vi "rszvl_core_global.vi"() -> ()   [LabVIEW 2014] (continued)
 BTO Get Modulation Accuracy of DEVM 99%:\nThis attribute reads the 99% of differential error vector magnitude (DEVM) in the Carrier Frequency Stability and Modulation Accuracy measurement.\n\nNote:\n\n(1) This command is only available with active Carrier Frequency Stability and Modulation\nAccuracy measurement.\n\n(18) BTO Get Carrier Frequency Stability Total Frequency Error Value:\nThis attribute reads the value of carrier frequency deviation of all packets in the Carrier Frequency Stability and Modulation Accuracy measurement.\n\nNote(s):\n\n(1) This command is only available with active Carrier Frequency Stability and Modulation Accuracy measurement\n\n(19) BTO Get Carrier Frequency Stability Block Frequency Error Value:\nThis attribute reads the frequency deviation of all blocks in the Carrier Frequency Stability and Modulation Accuracy measurement.\n\nNote(s):\n\n(1) This command is only available with active Carrier Frequency Stability and Modulation Accuracy measurement\n\n(20) BTO Get Carrier Frequency Stability Initial Frequency Error Value:\nThis attribute reads the combined frequency deviation of all packets and all blocks in the Carrier Frequency Stability and Modulation Accuracy measurement.\n\nNote(s):\n\n(1) This command is only available with active Carrier Frequency Stability and Modulation Accuracy measurement\n\n(21) BTO Get Diff Phase Encoding Tested Packets:\nThis attribute reads the number of tested packets in the Differential Phase Encoding measurement.\n\nNote(s):\n\n(1) This command is only available with active Carrier Frequency Stability and Modulation Accuracy measurement\n\n(22) BTO Get Diff Phase Encoding Passed Packets:\nThis attribute reads the number of passed packets in the Differential Phase Encoding measurement.\n\nNote(s):\n\n(1) This command is only available with active Carrier Frequency Stability and Modulation Accuracy measurement\n\n(23) BTO Get Diff Phase Encoding Bit Error Rate:\nThis attribute reads the bit error rate (BER) in the Differential Phase Encoding measurement.\n\nNote(s):\n\n(1) This command is only available with active Carrier Frequency Stability and Modulation Accuracy measurement\n\n(24) BTO Get Spurious Emissions Number Of Exceptions:\nThis attribute reads the number of results that exceeded the specified limits in the In–band Spurious Emissions measurement.\n\nNote: \n\n(1) This command is only available with active In–band Spurious Emissions measurement\n\n(25) BTO Get Spurious Emissions Adj 500 kHz:\nThis attribute reads the maximum power of the frequency band (500 kHz) of the TX channel in the In–band Spurious Emissions measurement.\n\nNote: \n\n(1) This command is only available with active In–band Spurious Emissions measurement\n\n(26) BTO Get Spurious Emissions Tx Channel Reference:\nThis attribute reads the TX channel reference power.\n\nNote: \n\n(1) This command is only available with active In–band Spurious Emissions measurement\n\n(27) BTO Get Relative Transmit Power:\nThis attribute reads the value average transmission power for the DPSK or GFSK sections of the packet in the Relative Transmission Power measurement. With a sweep count <= 1, the command returns the current value, irrespective of the parameter.\n\nNote: \n\n(1) This command is only available with active Relative Transmit Power measurement\n\n(28) BTO Get Relative Transmit Power Ratio:\nThis attribute reads the value of ratio of the transmission power for the GFSK and DPSK modulation in Relative Transmission Power measurement. With a sweep count <= 1, the command returns the current value, irrespective of the parameter.\n\nNote: \n\n(1) This command is only available with active Relative Transmit Power measurement", "Flags"={"OPC Wait"=FALSE, "Dont check status"=FALSE, "*WAI"=FALSE}, "Check Status Callback"=""}, {"Level"=3, "Descriptive Name"="BTO Get Output Power Peak", "Class Only"=FALSE, "Data Type"=1, "Access"=0, "Identifier"="RSZVL_ATTR_BTO_OPOW_PEAK", "Range Table"="", "Command"="CALC:BTO:OPOW?", "Read Callback"="", "Write Callback"="", "Range Callback"="", "Check Callback"="", "Rngtable Callback"="", "Coerce Callback"="", "User Callback"="", "Supported Models"="", "Instrument Options"="", "Repeated Capabilities"="", "Restricted Repeated Capabilities"="", "Help"="This attribute returns the peak value of the Output Power Measurement according to the BLUETOOTH standard.\n\nAvailable Repeated Capabilities:\nNone\n\nRemote-control command(s):\nCALCulate:BTOoth:OPOWer[:PEAK]?", "Flags"={"OPC Wait"=FALSE, "Dont check status"=FALSE, "*WAI"=FALSE}, "Check Status Callback"=""}, {"Level"=3, "Descriptive Name"="BTO Get Output Power Average", "Class Only"=FALSE, "Data Type"=1, "Access"=0, "Identifier"="RSZVL_ATTR_BTO_OPOW_AVER", "Range Table"="", "Command"="CALC:BTO:OPOW:AVER? {ModifMinMaxAver}", "Read Callback"="", "Write Callback"="", "Range Callback"="", "Check Callback"="", "Rngtable Callback"="", "Coerce Callback"="", "User Callback"="", "Supported Models"="", "Instrument Options"="", "Repeated Capabilities"="", "Restricted Repeated Capabilities"="", "Help"="This attribute reads the average value of the Output Power measurement according to the Bluetooth standard.\n\nAvailable Repeated Capabilities:\nModifMinMaxAver: Min,Max,Aver\r\n\nRemote-control command(s):\nCALCulate:BTOoth:OPOWer:AVERage? MINimum | MAXimum", "Flags"={"OPC Wait"=FALSE, "Dont check status"=FALSE, "*WAI"=FALSE}, "Check Status Callback"=""}, {"Level"=3, "Descriptive Name"="BTO Get Status", "Class Only"=FALSE, "Data Type"=0, "Access"=0, "Identifier"="RSZVL_ATTR_BTO_STAT", "Range Table"="", "Command"="CALC:BTO:STAT?", "Read Callback"="", "Write Callback"="", "Range Callback"="", "Check Callback"="", "Rngtable Callback"="", "Coerce Callback"="", "User Callback"="", "Supported Models"="", "Instrument Options"="", "Repeated Capabilities"="", "Restricted Repeated Capabilities"="", "Help"="This attribute queries the status of a preceeding measurement.\n\n0: PASS\n1: FAIL\n\nAvailable Repeated Capabilities:\nNone\n\nRemote-control command(s):\nCALCulate:BTOoth:STATus?", "Flags"={"OPC Wait"=FALSE, "Dont check status"=FALSE, "*WAI"=FALSE}, "Check Status Callback"=""}, {"Level"=3, "Descriptive Name"="BTO Get Number Of Exceptions", "Class Only"=FALSE, "Data Type"=0, "Access"=0, "Identifier"="RSZVL_ATTR_BTO_ACLR_EXC", "Range Table"="", "Command"="CALC:BTO:ACLR:EXC?", "Read Callback"="", "Write Callback"="", "Range Callback"="", "Check Callback"="", "Rngtable Callback"="", "Coerce Callback"="", "User Callback"="", "Supported Models"="", "Instrument Options"="", "Repeated Capabilities"="", "Restricted Repeated Capabilities"="", "Help"="This attribute returns the number of exceptions which occured during the adjacent channel\npower measurement according to the Bluetooth specification.\n\nAvailable Repeated Capabilities:\nNone\n\nRemote-control command(s):\nCALCulate:BTOoth:ACLR:EXCeptions?", "Flags"={"OPC Wait"=FALSE, "Dont check status"=FALSE, "*WAI"=FALSE}, "Check Status Callback"=""}, {"Level"=3, "Descriptive Name"="BTO Get Average Frequency Deviation", "Class Only"=FALSE, "Data Type"=1, "Access"=0, "Identifier"="RSZVL_ATTR_BTO_MCH_DF_AVER", "Range Table"="", "Command"="CALC:BTO:MCH:DF{Frequency}:AVER? {ModifMinMaxAver}", "Read Callback"="", "Write Callback"="", "Range Callback"="", "Check Callback"="", "Rngtable Callback"="", "Coerce Callback"="", "User Callback"="", "Supported Models"="", "Instrument Options"="", "Repeated Capabilities"="", "Restricted Repeated Capabilities"="", "Help"="This attribute returns the value of average frequency deviation for varying bit patterns of the payload.\n\nAvailable Repeated Capabilities:\nFrequency: F1,F2\r\nModifMinMaxAver: Min,Max,Aver\r\n\nRemote-control command(s):\nCALCulate:BTOoth:MCHar:DF<1|2>:AVERage? MINimum | MAXimum", "Flags"={"OPC Wait"=FALSE, "Dont check status"=FALSE, "*WAI"=FALSE}, "Check Status Callback"=""}, {"Level"=3, "Descriptive Name"="BTO Get Maximum Frequency Deviation Value", "Class Only"=FALSE, "Data Type"=1, "Access"=0, "Identifier"="RSZVL_ATTR_BTO_MCH_DF_MAX", "Range Table"="", "Command"="CALC:BTO:MCH:DF{Frequency}:MAX? {ModifMinMaxAver}", "Read Callback"="", "Write Callback"="", "Range Callback"="", "Check Callback"="", "Rngtable Callback"="", "Coerce Callback"="", "User Callback"="", "Supported Models"="", "Instrument Options"="", "Repeated Capabilities"="", "Restricted Repeated Capabilities"="", "Help"="This attribute returns the value of maximum frequency deviation for different bit patterns of the payload.\n\nAvailable Repeated Capabilities:\nFrequency: F1,F2\r\nModifMinMaxAver: Min,Max,Aver\r\n\nRemote-control command(s):\nCALCulate:BTOoth:MCHar:DF<1|2>:MAXimum? MINimum | MAXimum | AVERage", "Flags"={"OPC Wait"=FALSE, "Dont check status"=FALSE, "*WAI"=FALSE}, "Check Status Callback"=""}, {"Level"=3, "Descriptive Name"="BTO Get Ratio Of Average Frequency Deviations Value", "Class Only"=FALSE, "Data Type"=1, "Access"=0, "Identifier"="RSZVL_ATTR_BTO_MCH_RAT", "Range Table"="", "Command"="CALC:BTO:MCH:RAT? {ModifMinMaxAver}", "Read Callback"="", "Write Callback"="", "Range Callback"="", "Check Callback"="", "Rngtable Callback"="", "Coerce Callback"="", "User Callback"="", "Supported Models"="", "Instrument Options"="", "Repeated Capabilities"="", "Restricted Repeated Capabilities"="", "Help"="This attribute returns the value of ratio of the average frequency deviations for varying bit patterns of the payload.\n\nAvailable Repeated Capabilities:\nModifMinMaxAver: Min,Max,Aver\r\n\nRemote-control command(s):\nCALCulate:BTOoth:MCHar:RATio? MINimum | MAXimum | AVERage", "Flags"={"OPC Wait"=FALSE, "Dont check status"=FALSE, "*WAI"=FALSE}, "Check Status Callback"=""}, {"Level"=3, "Descriptive Name"="BTO Get Percentage Deviation", "Class Only"=FALSE, "Data Type"=1, "Access"=0, "Identifier"="RSZVL_ATTR_BTO_MCH_DF2_PERC", "Range Table"="", "Command"="CALC:BTO:MCH:DF2:PERC?", "Read Callback"="", "Write Callback"="", "Range Callback"="", "Check Callback"="", "Rngtable Callback"="", "Coerce Callback"="", "User Callback"="", "Supported Models"="", "Instrument Options"="", "Repeated Capabilities"="", "Restricted Repeated Capabilities"="", "Help"="This attribute returns the percentage of measurements of the frequency deviation.\n\nAvailable Repeated Capabilities:\nNone\n\nRemote-control command(s):\nCALCulate:BTOoth:MCHar:DF2:PERCent?", "Flags"={"OPC Wait"=FALSE, "Dont check status"=FALSE, "*WAI"=FALSE}, "Check Status Callback"=""}, {"Level"=3, "Descriptive Name"="BTO Get Initial Carrier Frequency Tolerance Value", "Class Only"=FALSE, "Data Type"=1, "Access"=0, "Identifier"="RSZVL_ATTR_BTO_ICFT", "Range Table"="", "Command"="CALC:BTO:ICFT? {ModifMinMaxAver}", "Read Callback"="", "Write Callback"="", "Range Callback"="", "Check Callback"="", "Rngtable Callback"="", "Coerce Callback"="", "User Callback"="", "Supported Models"="", "Instrument Options"="", "Repeated Capabilities"="", "Restricted Repeated Capabilities"="", "Help"="This attribute returns value of the Initial Carrier Frequency Tolerance.\n\nNote(s):\n(1) This command is only available with active Initial Carrier Frequency Tolerance measurement (command CONF:BTO:MEAS ICFT). With all other measurements this command will lead to a query error.\n\nAvailable Repeated Capabilities:\nModifMinMaxAver: Min,Max,Aver\r\n\nRemote-control command(s):\nCALCulate:BTOoth:ICFTolerance? MINimum | MAXimum | AVERage", "Flags"={"OPC Wait"=FALSE, "Dont check status"=FALSE, "*WAI"=FALSE}, "Check Status Callback"=""}, {"Level"=3, "Descriptive Name"="BTO Get Maximum Carrier Frequency Drift", "Class Only"=FALSE, "Data Type"=1, "Access"=0, "Identifier"="RSZVL_ATTR_BTO_CFDR_MAX", "Range Table"="", "Command"="CALC:BTO:CFDR?", "Read Callback"="", "Write Callback"="", "Range Callback"="", "Check Callback"="", "Rngtable Callback"="", "Coerce Callback"="", "User Callback"="", "Supported Models"="", "Instrument Options"="", "Repeated Capabilities"="", "Restricted Repeated Capabilities"="", "Help"="This attribute returns the maximum Carrier Frequency Drift.\n\nNote(s):\n(1) This command is only available with active Carrier Frequency Drift measurement (command CONF:BTO:MEAS CFDR). With all other measurements this command will lead to a query error.\n\nAvailable Repeated Capabilities:\nNone\n\nRemote-control command(s):\nCALCulate:BTOoth:CFDRift[:MAXimum]?", "Flags"={"OPC Wait"=FALSE, "Dont check status"=FALSE, "*WAI"=FALSE}, "Check Status Callback"=""}, {"Level"=3, "Descriptive Name"="BTO Get Carrier Frequency Drift", "Class Only"=FALSE, "Data Type"=1, "Access"=0, "Identifier"="RSZVL_ATTR_BTO_CFDR_RATE", "Range Table"="", "Command"="CALC:BTO:CFDR:RATE?", "Read Callback"="", "Write Callback"="", "Range Callback"="", "Check Callback"="", "Rngtable Callback"="", "Coerce Callback"="", "User Callback"="", "Supported Models"="", "Instrument Options"="", "Repeated Capabilities"="", "Restricted Repeated Capabilities"="", "Help"="This attribute returns the maximum Carrier Frequency Drift per 50 ms.\n\nNote(s):\n(1) This command is only available with active Carrier Frequency Drift measurement (command CONF:BTO:MEAS CFDR). With all other measurements this command will lead to a query error.\n\nAvailable Repeated Capabilities:\nNone\n\nRemote-control command(s):\nCALCulate:BTOoth:CFDRift:RATE?", "Flags"={"OPC Wait"=FALSE, "Dont check status"=FALSE, "*WAI"=FALSE}, "Check Status Callback"=""}, {"Level"=3, "Descriptive Name"="BTO Get Packet Length", "Class Only"=FALSE, "Data Type"=0, "Access"=0, "Identifier"="RSZVL_ATTR_BTO_PLEN", "Range Table"="", "Command"="CALC:BTO:PLEN?", "Read Callback"="", "Write Callback"="", "Range Callback"="", "Check Callback"="", "Rngtable Callback"="", "Coerce Callback"="", "User Callback"="", "Supported Models"="", "Instrument Options"="", "Repeated Capabilities"="", "Restricted Repeated Capabilities"="", "Help"="This attribute returns the length of the packet analyzed by the preceeding measurement.\n\nAvailable Repeated Capabilities:\nNone\n\nRemote-control command(s):\nCALCulate:BTOoth:PLENgth?", "Flags"={"OPC Wait"=FALSE, "Dont check status"=FALSE, "*WAI"=FALSE}, "Check Status Callback"=""}, {"Level"=3, "Descriptive Name"="BTO Get Packet Type", "Class Only"=FALSE, "Data Type"=0, "Access"=0, "Identifier"="RSZVL_ATTR_BTO_PTYP", "Range Table"="rszvl_rngBtoPtype", "Command"="CALC:BTO:PTYP?", "Read Callback"="", "Write Callback"="", "Range Callback"="", "Check Callback"="", "Rngtable Callback"="", "Coerce Callback"="", "User Callback"="", "Supported Models"="", "Instrument Options"="", "Repeated Capabilities"="", "Restricted Repeated Capabilities"="", "Help"="This attribute returns the type of the packet analyzed by a preceeding measurement.\n\nAvailable Repeated Capabilities:\nNone\n\nRemote-control command(s):\nCALCulate:BTOoth:PTYPe?", "Flags"={"OPC Wait"=FALSE, "Dont check status"=FALSE, "*WAI"=FALSE}, "Check Status Callback"=""}, {"Level"=3, "Descriptive Name"="BTO Get Measured Block", "Class Only"=FALSE, "Data Type"=0, "Access"=0, "Identifier"="RSZVL_ATTR_BTO_CFST_BLOCK_COUNT_VALUE", "Range Table"="", "Command"="CALC:BTO:CFST:COUN?", "Read Callback"="", "Write Callback"="", "Range Callback"="", "Check Callback"="", "Rngtable Callback"="", "Coerce Callback"="", "User Callback"="", "Supported Models"="", "Instrument Options"="", "Repeated Capabilities"="", "Restricted Repeated Capabilities"="", "Help"="This attribute reads the number of measured blocks during or after a measurement.\n\nNote:\n\n(1) This command is only available with active Carrier Frequency Stability and Modulation\nAccuracy measurement.\n\nAvailable Repeated Capabilities:\nNone\n\nRemote-control command(s):\nCALCulate<1|2>:BTOoth:CFSTability:COUNt?", "Flags"={"OPC Wait"=FALSE, "Dont check status"=FALSE, "*WAI"=FALSE}, "Check Status Callback"=""}, {"Level"=3, "Descriptive Name"="BTO Get Modulation Accuracy of DEVM RMS", "Class Only"=FALSE, "Data Type"=1, "Access"=0, "Identifier"="RSZVL_ATTR_BTO_CFST_DEVM_RMS", "Range Table"="", "Command"="CALC:BTO:CFST:DEVM:RMS? {ModifMinMaxAver}", "Read Callback"="", "Write Callback"="", "Range Callback"="", "Check Callback"="", "Rngtable Callback"="", "Coerce Callback"="", "User Callback"="", "Supported Models"="", "Instrument Options"="", "Repeated Capabilities"="", "Restricted Repeated Capabilities"="", "Help"="This attribute reads the RMAS of differential error vector magnitude (DEVM) in the Carrier Frequency Stability and Modulation Accuracy measurement.\n\nNote:\n\n(1) This command is only available with active Carrier Frequency Stability and Modulation\nAccuracy measurement.\n\nAvailable Repeated Capabilities:\nModifMinMaxAver: Min,Max,Aver\r\n\nRemote-control command(s):\nCALCulate<1|2>:BTOoth:CFSTability:DEVM:[RMS]? MINimum | MAXimum | AVERage", "Flags"={"OPC Wait"=FALSE, "Dont check status"=FALSE, "*WAI"=FALSE}, "Check Status Callback"=""}, {"Level"=3, "Descriptive Name"="BTO Get Modulation Accuracy of DEVM Peak", "Class Only"=FALSE, "Data Type"=1, "Access"=0, "Identifier"="RSZVL_ATTR_BTO_CFST_DEVM_PEAK", "Range Table"="", "Command"="CALC:BTO:CFST:DEVM:PEAK?", "Read Callback"="", "Write Callback"="", "Range Callback"="", "Check Callback"="", "Rngtable Callback"="", "Coerce Callback"="", "User Callback"="", "Supported Models"="", "Instrument Options"="", "Repeated Capabilities"="", "Restricted Repeated Capabilities"="", "Help"="This attribute reads the Peak of differential error vector magnitude (DEVM) in the Carrier Frequency Stability and Modulation Accuracy measurement.\n\nNote:\n\n(1) This command is only available with active Carrier Frequency Stability and Modulation\nAccuracy measurement.\n\nAvailable Repeated Capabilities:\nNone\n\nRemote-control command(s):\nCALCulate<1|2>:BTOoth:CFSTability:DEVM:PEAK?", "Flags"={"OPC Wait"=FALSE, "Dont check status"=FALSE, "*WAI"=FALSE}, "Check Status Callback"=""}, {"Level"=3, "Descriptive Name"="BTO Get Modulation Accuracy of DEVM 99%", "Class Only"=FALSE, "Data Type"=1, "Access"=0, "Identifier"="RSZVL_ATTR_BTO_CFST_DEVM_99PCT", "Range Table"="", "Command"="CALC:BTO:CFST:DEVM:D99P?", "Read Callback"="", "Write Callback"="", "Range Callback"="", "Check Callback"="", "Rngtable Callback"="", "Coerce Callback"="", "User Callback"="", "Supported Models"="", "Instrument Options"="", "Repeated Capabilities"="", "Restricted Repeated Capabilities"="", "Help"="This attribute reads the 99% of differential error vector magnitude (DEVM) in the Carrier Frequency Stability and Modulation Accuracy measurement.\n\nNote:\n\n(1) This command is only available with active Carrier Frequency Stability and Modulation\nAccuracy measurement.\n\nAvailable Repeated Capabilities:\nNone\n\nRemote-control command(s):\nCALCulate<1|2>:BTOoth:CFSTability:DEVM:D99Pct?", "Flags"={"OPC Wait"=FALSE, "Dont check status"=FALSE, "*WAI"=FALSE}, "Check Status Callback"=""}, {"Level"=3, "Descriptive Name"="BTO Get Carrier Frequency Stability Total Frequency Error Value", "Class Only"=FALSE, "Data Type"=1, "Access"=0, "Identifier"="RSZVL_ATTR_BTO_CFST_FERR_TOTAL", "Range Table"="", "Command"="CALC:BTO:CFST:FERR? {ModifMinMaxAver}", "Read Callback"="", "Write Callback"="", "Range Callback"="", "Check Callback"="", "Rngtable Callback"="", "Coerce Callback"="", "User Callback"="", "Supported Models"="", "Instrument Options"="", "Repeated Capabilities"="", "Restricted Repeated Capabilities"="", "Help"="This attribute reads the value of carrier frequency deviation of all packets in the Carrier Frequency Stability and Modulation Accuracy measurement.\n\nNote(s):\n\n(1) This command is only available with active Carrier Frequency Stability and Modulation Accuracy measurement\n\nAvailable Repeated Capabilities:\nModifMinMaxAver: Min,Max,Aver\r\n\nRemote-control command(s):\nCALCulate<1|2>:BTOoth:CFSTability:FERRor:[TOTal]? MINimum | MAXimum | AVERage", "Flags"={"OPC Wait"=FALSE, "Dont check status"=FALSE, "*WAI"=FALSE}, "Check Status Callback"=""}, {"Level"=3, "Descriptive Name"="BTO Get Carrier Frequency Stability Block Frequency Error Value", "Class Only"=FALSE, "Data Type"=1, "Access"=0, "Identifier"="RSZVL_ATTR_BTO_CFST_FERR_BLOCK", "Range Table"="", "Command"="CALC:BTO:CFST:FERR:BLOC? {ModifMinMaxAver}", "Read Callback"="", "Write Callback"="", "Range Callback"="", "Check Callback"="", "Rngtable Callback"="", "Coerce Callback"="", "User Callback"="", "Supported Models"="", "Instrument Options"="", "Repeated Capabilities"="", "Restricted Repeated Capabilities"="", "Help"="This attribute reads the frequency deviation of all blocks in the Carrier Frequency Stability and Modulation Accuracy measurement.\n\nNote(s):\n\n(1) This command is only available with active Carrier Frequency Stability and Modulation Accuracy measurement\n\nAvailable Repeated Capabilities:\nModifMinMaxAver: Min,Max,Aver\r\n\nRemote-control command(s):\nCALCulate<1|2>:BTOoth:CFSTability:FERRor:BLOCk? MINimum | MAXimum | AVERage", "Flags"={"OPC Wait"=FALSE, "Dont check status"=FALSE, "*WAI"=FALSE}, "Check Status Callback"=""}, {"Level"=3, "Descriptive Name"="BTO Get Carrier Frequency Stability Initial Frequency Error Value", "Class Only"=FALSE, "Data Type"=1, "Access"=0, "Identifier"="RSZVL_ATTR_BTO_CFST_FERR_INITIAL", "Range Table"="", "Command"="CALC:BTO:CFST:FERR:INIT? {ModifMinMaxAver}", "Read Callback"="", "Write Callback"="", "Range Callback"="", "Check Callback"="", "Rngtable Callback"="", "Coerce Callback"="", "User Callback"="", "Supported Models"="", "Instrument Options"="", "Repeated Capabilities"="", "Restricted Repeated Capabilities"="", "Help"="This attribute reads the combined frequency deviation of all packets and all blocks in the Carrier Frequency Stability and Modulation Accuracy measurement.\n\nNote(s):\n\n(1) This command is only available with active Carrier Frequency Stability and Modulation Accuracy measurement\n\nAvailable Repeated Capabilities:\nModifMinMaxAver: Min,Max,Aver\r\n\nRemote-control command(s):\nCALCulate<1|2>:BTOoth:CFSTability:FERRor:INITial? MINimum | MAXimum | AVERage", "Flags"={"OPC Wait"=FALSE, "Dont check status"=FALSE, "*WAI"=FALSE}, "Check Status Callback"=""}, {"Level"=3, "Descriptive Name"="BTO Get Diff Phase Encoding Tested Packets", "Class Only"=FALSE, "Data Type"=0, "Access"=0, "Identifier"="RSZVL_ATTR_BTO_DPEN_PACKETS", "Range Table"="", "Command"="CALC:BTO:DPEN?", "Read Callback"="", "Write Callback"="", "Range Callback"="", "Check Callback"="", "Rngtable Callback"="", "Coerce Callback"="", "User Callback"="", "Supported Models"="", "Instrument Options"="", "Repeated Capabilities"="", "Restricted Repeated Capabilities"="", "Help"="This attribute reads the number of tested packets in the Differential Phase Encoding measurement.\n\nNote(s):\n\n(1) This command is only available with active Carrier Frequency Stability and Modulation Accuracy measurement\n\nAvailable Repeated Capabilities:\nNone\n\nRemote-control command(s):\nCALCulate<1|2>:BTOoth:DPENcoding:[TOTal]?", "Flags"={"OPC Wait"=FALSE, "Dont check status"=FALSE, "*WAI"=FALSE}, "Check Status Callback"=""}, {"Level"=3, "Descriptive Name"="BTO Get Diff Phase Encoding Passed Packets", "Class Only"=FALSE, "Data Type"=0, "Access"=0, "Identifier"="RSZVL_ATTR_BTO_DPEN_PACKETS_PASSED", "Range Table"="", "Command"="CALC:BTO:DPEN:NERR?", "Read Callback"="", "Write Callback"="", "Range Callback"="", "Check Callback"="", "Rngtable Callback"="", "Coerce Callback"="", "User Callback"="", "Supported Models"="", "Instrument Options"="", "Repeated Capabilities"="", "Restricted Repeated Capabilities"="", "Help"="This attribute reads the number of passed packets in the Differential Phase Encoding measurement.\n\nNote(s):\n\n(1) This command is only available with active Carrier Frequency Stability and Modulation Accuracy measurement\n\nAvailable Repeated Capabilities:\nNone\n\nRemote-control command(s):\nCALCulate<1|2>:BTOoth:DPENcoding:NERRor?", "Flags"={"OPC Wait"=FALSE, "Dont check status"=FALSE, "*WAI"=FALSE}, "Check Status Callback"=""}, {"Level"=3, "Descriptive Name"="BTO Get Diff Phase Encoding Bit Error Rate", "Class Only"=FALSE, "Data Type"=0, "Access"=0, "Identifier"="RSZVL_ATTR_BTO_DPEN_BER", "Range Table"="", "Command"="CALC:BTO:DPEN:BER?", "Read Callback"="", "Write Callback"="", "Range Callback"="", "Check Callback"="", "Rngtable Callback"="", "Coerce Callback"="", "User Callback"="", "Supported Models"="", "Instrument Options"="", "Repeated Capabilities"="", "Restricted Repeated Capabilities"="", "Help"="This attribute reads the bit error rate (BER) in the Differential Phase Encoding measurement.\n\nNote(s):\n\n(1) This command is only available with active Carrier Frequency Stability and Modulation Accuracy measurement\n\nAvailable Repeated Capabilities:\nNone\n\nRemote-control command(s):\nCALCulate<1|2>:BTOoth:DPENcoding:BER?", "Flags"={"OPC Wait"=FALSE, "Dont check status"=FALSE, "*WAI"=FALSE}, "Check Status Callback"=""}, {"Level"=3, "Descriptive Name"="BTO Get Spurious Emissions Number Of Exceptions", "Class Only"=FALSE, "Data Type"=0, "Access"=0, "Identifier"="RSZVL_ATTR_BTO_IBS_EXC", "Range Table"="", "Command"="CALC:BTO:IBS:EXC?", "Read Callback"="", "Write Callback"="", "Range Callback"="", "Check Callback"="", "Rngtable Callback"="", "Coerce Callback"="", "User Callback"="", "Supported Models"="", "Instrument Options"="", "Repeated Capabilities"="", "Restricted Repeated Capabilities"="", "Help"="This attribute reads the number of results that exceeded the specified limits in the In–band Spurious Emissions measurement.\n\nNote: \n\n(1) This command is only available with active In–band Spurious Emissions measurement\n\nAvailable Repeated Capabilities:\nNone\n\nRemote-control command(s):\nCALCulate<1|2>:BTOoth:IBSemissions:EXCeptions?", "Flags"={"OPC Wait"=FALSE, "Dont check status"=FALSE, "*WAI"=FALSE}, "Check Status Callback"=""}, {"Level"=3, "Descriptive Name"="BTO Get Spurious Emissions Adj 500 kHz", "Class Only"=FALSE, "Data Type"=1, "Access"=0, "Identifier"="RSZVL_ATTR_BTO_IBS_HADJ", "Range Table"="", "Command"="CALC:BTO:IBS:HADJ? {ModifLowUpp}", "Read Callback"="", "Write Callback"="", "Range Callback"="", "Check Callback"="", "Rngtable Callback"="", "Coerce Callback"="", "User Callback"="", "Supported Models"="", "Instrument Options"="", "Repeated Capabilities"="", "Restricted Repeated Capabilities"="", "Help"="This attribute reads the maximum power of the frequency band (500 kHz) of the TX channel in the In–band Spurious Emissions measurement.\n\nNote: \n\n(1) This command is only available with active In–band Spurious Emissions measurement\n\nAvailable Repeated Capabilities:\nModifLowUpp: Low,Upp\r\n\nRemote-control command(s):\nCALCulate<1|2>:BTOoth:IBSemissions:HADJacent? UPPer | LOWer", "Flags"={"OPC Wait"=FALSE, "Dont check status"=FALSE, "*WAI"=FALSE}, "Check Status Callback"=""}, {"Level"=3, "Descriptive Name"="BTO Get Spurious Emissions Tx Channel Reference", "Class Only"=FALSE, "Data Type"=1, "Access"=0, "Identifier"="RSZVL_ATTR_BTO_IBS_TXCHANNEL", "Range Table"="", "Command"="CALC:BTO:IBS:TXR?", "Read Callback"="", "Write Callback"="", "Range Callback"="", "Check Callback"="", "Rngtable Callback"="", "Coerce Callback"="", "User Callback"="", "Supported Models"="", "Instrument Options"="", "Repeated Capabilities"="", "Restricted Repeated Capabilities"="", "Help"="This attribute reads the TX channel reference power.\n\nNote: \n\n(1) This command is only available with active In–band Spurious Emissions measurement\n\nAvailable Repeated Capabilities:\nNone\n\nRemote-control command(s):\nCALCulate<1|2>:BTOoth:IBSemissions:TXReference?", "Flags"={"OPC Wait"=FALSE, "Dont check status"=FALSE, "*WAI"=FALSE}, "Check Status Callback"=""}, {"Level"=3, "Descriptive Name"="BTO Get Relative Transmit Power", "Class Only"=FALSE, "Data Type"=1, "Access"=0, "Identifier"="RSZVL_ATTR_BTO_RTP", "Range Table"="", "Command"="CALC:BTO:RTP:{BtoRtpPacketSection}? {ModifMinMaxAver}", "Read Callback"="", "Write Callback"="", "Range Callback"="", "Check Callback"="", "Rngtable Callback"="", "Coerce Callback"="", "User Callback"="", "Supported Models"="", "Instrument Options"="", "Repeated Capabilities"="", "Restricted Repeated Capabilities"="", "Help"="This attribute reads the value average transmission power for the DPSK or GFSK sections of the packet in the Relative Transmission Power measurement. With a sweep count <= 1, the command returns the current value, irrespective of the parameter.\n\nNote: \n\n(1) This command is only available with active Relative Transmit Power measurement\n\nAvailable Repeated Capabilities:\nBtoRtpPacketSection: SECTION_GFSK,SECTION_DPSK\r\nModifMinMaxAver: Min,Max,Aver\r\n\nRemote-control command(s):\nCALCulate<1|2>:BTOoth:RTPower:[DPSK]? MINimum | MAXimum | AVERage", "Flags"={"OPC Wait"=FALSE, "Dont check status"=FALSE, "*WAI"=FALSE}, "Check Status Callback"=""}, {"Level"=3, "Descriptive Name"="BTO Get Relative Transmit Power Ratio", "Class Only"=FALSE, "Data Type"=1, "Access"=0, "Identifier"="RSZVL_ATTR_BTO_RTP_RATIO", "Range Table"="", "Command"="CALC:BTO:RTP:RAT? {ModifMinMaxAver}", "Read Callback"="", "Write Callback"="", "Range Callback"="", "Check Callback"="", "Rngtable Callback"="", "Coerce Callback"="", "User Callback"="", "Supported Models"="", "Instrument Options"="", "Repeated Capabilities"="", "Restricted Repeated Capabilities"="", "Help"="This attribute reads the value of ratio of the transmission power for the GFSK and DPSK modulation in Relative Transmission Power measurement. With a sweep count <= 1, the command returns the current value, irrespective of the parameter.\n\nNote: \n\n(1) This command is only available with active Relative Transmit Power measurement\n\nAvailable Repeated Capabilities:\nModifMinMaxAver: Min,Max,Aver\r\n\nRemote-control command(s):\nCALCulate<1|2>:BTOoth:RTPower:RATio? MINimum | MAXimum | AVERage", "Flags"={"OPC Wait"=FALSE, "Dont check status"=FALSE, "*WAI"=FALSE}, "Check Status Callback"=""}, {"Level"=1, "Descriptive Name"="K9 - Power Meter", "Class Only"=TRUE, "Data Type"=0, "Access"=0, "Identifier"="", "Range Table"="", "Command"="", "Read Callback"="", "Write Callback"="", "Range Callback"="", "Check Callback"="", "Rngtable Callback"="", "Coerce Callback"="", "User Callback"="", "Supported Models"="", "Instrument Options"="", "Repeated Capabilities"="", "Restricted Repeated Capabilities"="", "Help"="(1) Settings (Class):\n(1) PWM Reference value:\nThis attribute sets the reference value for relative measurements.\n\n(2) PWM Measure To Reference:\nThis attribute accepts the current result as a reference value for relative measurements.\n\n(3) PWM Frequency:\nThis attribute sets the frequency of the power sensor.\nThe limit values fmin and fmax are set by the power sensor that is connected.\n\n(4) PWM Measurement Time:\nThis attribute determines the measurement time of the power sensor.\n\n(5) PWM Frequency Coupling:\nThis attribute sets the coupling for the frequency of the power sensor.\n\n(6) PWM Zero:\nThis attribute zeroes the power sensor.\n\nNote:\n(1) *WAI is send after command\n\n(7) PWM Absolute Unit:\nThis attribute selects the unit for absolute measurements with a power sensor.\n\n(8) PWM Relative Units:\nThis attribute selects the unit for relative measurements with a power sensor.\n\n(9) PWM Power Meter State:\nThis attribute switches measurements with a power sensor on or off.\n\n\n\n(2) Display (Class):\n(1) PWM Result Display:\nThis attribute switches bargraph display on or off for measurements with a power sensor. If bargraph display is switched off, the measurement value appears in the Marker Info field.\n\n(2) PWM Rel/Abs Display:\nThis attribute switches between relative and absolute display of the result.\n\n\n\n(3) Results (Class):\n(1) PWM Read Result:\nThis attribute triggers a measurement with the power sensor and then outputs the result.\n\n(2) PWM Fetch Result:\nThis attribute outputs the result of the power sensor.", "Flags"={"OPC Wait"=FALSE, "Dont check status"=FALSE, "*WAI"=FALSE}, "Check Status Callback"=""}, {"Level"=2, "Descriptive Name"="Settings", "Class Only"=TRUE, "Data Type"=0, "Access"=0, "Identifier"="", "Range Table"="", "Command"="", "Read Callback"="", "Write Callback"="", "Range Callback"="", "Check Callback"="", "Rngtable Callback"="", "Coerce Callback"="", "User Callback"="", "Supported Models"="", "Instrument Options"="", "Repeated Capabilities"="", "Restricted Repeated Capabilities"="", "Help"="(1) PWM Reference value:\nThis attribute sets the reference value for relative measurements.\n\n(2) PWM Measure To Reference:\nThis attribute accepts the current result as a reference value for relative measurements.\n\n(3) PWM Frequency:\nThis attribute sets the frequency of the power sensor.\nThe limit values fmin and fmax are set by the power sensor that is connected.\n\n(4) PWM Measurement Time:\nThis attribute determines the measurement time of the power sensor.\n\n(5) PWM Frequency Coupling:\nThis attribute sets the coupling for the frequency of the power sensor.\n\n(6) PWM Zero:\nThis attribute zeroes the power sensor.\n\nNote:\n(1) *WAI is send after command\n\n(7) PWM Absolute Unit:\nThis attribute selects the unit for absolute measurements with a power sensor.\n\n(8) PWM Relative Units:\nThis attribute selects the unit for relative measurements with a power sensor.\n\n(9) PWM Power Meter State:\nThis attribute switches measurements with a power sensor on or off.", "Flags"={"OPC Wait"=FALSE, "Dont check status"=FALSE, "*WAI"=FALSE}, "Check Status Callback"=""}, {"Level"=3, "Descriptive Name"="PWM Reference value", "Class Only"=FALSE, "Data Type"=1, "Access"=2, "Identifier"="RSZVL_ATTR_PMET_REL", "Range Table"="rszvl_rngRefLevel", "Command"="CALC:PMET:REL", "Read Callback"="", "Write Callback"="", "Range Callback"="", "Check Callback"="", "Rngtable Callback"="", "Coerce Callback"="", "User Callback"="", "Supported Models"="", "Instrument Options"="", "Repeated Capabilities"="", "Restricted Repeated Capabilities"="", "Help"="This attribute sets the reference value for relative measurements.\n\nAvailable Repeated Capabilities:\nNone\n\nRemote-control command(s):\nCALCulate<1|2>:PMETer:RELative[:MAGNitude]", "Flags"={"OPC Wait"=FALSE, "Dont check status"=FALSE, "*WAI"=FALSE}, "Check Status Callback"=""}, {"Level"=3, "Descriptive Name"="PWM Measure To Reference", "Class Only"=FALSE, "Data Type"=4, "Access"=1, "Identifier"="RSZVL_ATTR_PMET_REL_AUTO", "Range Table"="", "Command"="CALC:PMET:REL:AUTO ONCE", "Read Callback"="", "Write Callback"="", "Range Callback"="", "Check Callback"="", "Rngtable Callback"="", "Coerce Callback"="", "User Callback"="", "Supported Models"="", "Instrument Options"="", "Repeated Capabilities"="", "Restricted Repeated Capabilities"="", "Help"="This attribute accepts the current result as a reference value for relative measurements.\n\nAvailable Repeated Capabilities:\nNone\n\nRemote-control command(s):\nCALCulate<1|2>:PMETer:RELative[:MAGNitude]:AUTO ONCE", "Flags"={"OPC Wait"=TRUE, "Dont check status"=FALSE, "*WAI"=FALSE}, "Check Status Callback"=""}, {"Level"=3, "Descriptive Name"="PWM Frequency", "Class Only"=FALSE, "Data Type"=1, "Access"=2, "Identifier"="RSZVL_ATTR_PMET_FREQ", "Range Table"="", "Command"="SENS:PMET:FREQ", "Read Callback"="", "Write Callback"="", "Range Callback"="", "Check Callback"="", "Rngtable Callback"="", "Coerce Callback"="", "User Callback"="", "Supported Models"="", "Instrument Options"="", "Repeated Capabilities"="", "Restricted Repeated Capabilities"="", "Help"="This attribute sets the frequency of the power sensor.\nThe limit values fmin and fmax are set by the power sensor that is connected.\n\nAvailable Repeated Capabilities:\nNone\n\nRemote-control command(s):\n[SENSe<1|2>:]PMETer:FREQuency", "Flags"={"OPC Wait"=FALSE, "Dont check status"=FALSE, "*WAI"=FALSE}, "Check Status Callback"=""}, {"Level"=3, "Descriptive Name"="PWM Measurement Time", "Class Only"=FALSE, "Data Type"=0, "Access"=2, "Identifier"="RSZVL_ATTR_PMET_MEAS_TIME", "Range Table"="rszvl_rngPmetMeasTime", "Command"="SENS:PMET:MTIM", "Read Callback"="", "Write Callback"="", "Range Callback"="", "Check Callback"="", "Rngtable Callback"="", "Coerce Callback"="", "User Callback"="", "Supported Models"="", "Instrument Options"="", "Repeated Capabilities"="", "Restricted Repeated Capabilities"="", "Help"="This attribute determines the measurement time of the power sensor.\n\nAvailable Repeated Capabilities:\nNone\n\nRemote-control command(s):\n[SENSe<1|2>:]PMETer:MTIMe SHORt | NORMal | LONG", "Flags"={"OPC Wait"=TRUE, "Dont check status"=FALSE, "*WAI"=FALSE}, "Check Status Callback"=""}, {"Level"=3, "Descriptive Name"="PWM Frequency Coupling", "Class Only"=FALSE, "Data Type"=0, "Access"=2, "Identifier"="RSZVL_ATTR_PMET_COUPLING", "Range Table"="rszvl_rngPmetCoupling", "Command"="SENS:PMET:FREQ:LINK", "Read Callback"="", "Write Callback"="", "Range Callback"="", "Check Callback"="", "Rngtable Callback"="", "Coerce Callback"="", "User Callback"="", "Supported Models"="", "Instrument Options"="", "Repeated Capabilities"="", "Restricted Repeated Capabilities"="", "Help"="This attribute sets the coupling for the frequency of the power sensor.\n\nAvailable Repeated Capabilities:\nNone\n\nRemote-control command(s):\n[SENSe<1|2>:]PMETer:FREQuency:LINK CENTer | MARKer1 | OFF", "Flags"={"OPC Wait"=FALSE, "Dont check status"=FALSE, "*WAI"=FALSE}, "Check Status Callback"=""}, {"Level"=3, "Descriptive Name"="PWM Zero", "Class Only"=FALSE, "Data Type"=4, "Access"=1, "Identifier"="RSZVL_ATTR_PMET_ZERO", "Range Table"="", "Command"=":CAL:PMET:ZERO:AUTO ONCE;*WAI", "Read Callback"="", "Write Callback"="", "Range Callback"="", "Check Callback"="", "Rngtable Callback"="", "Coerce Callback"="", "User Callback"="", "Supported Models"="", "Instrument Options"="", "Repeated Capabilities"="", "Restricted Repeated Capabilities"="", "Help"="This attribute zeroes the power sensor.\n\nNote:\n(1) *WAI is send after command\n\nAvailable Repeated Capabilities:\nNone\n\nRemote-control command(s):\nCALibration:PMETer:ZERO:AUTO ONCE", "Flags"={"OPC Wait"=FALSE, "Dont check status"=FALSE, "*WAI"=FALSE}, "Check Status Callback"=""}, {"Level"=3, "Descriptive Name"="PWM Absolute Unit", "Class Only"=FALSE, "Data Type"=0, "Access"=2, "Identifier"="RSZVL_ATTR_PMET_UNIT_ABS", "Range Table"="rszvl_rngPmetUnitAbs", "Command"="UNIT:PMET:POW", "Read Callback"="", "Write Callback"="", "Range Callback"="", "Check Callback"="", "Rngtable Callback"="", "Coerce Callback"="", "User Callback"="", "Supported Models"="", "Instrument Options"="", "Repeated Capabilities"="", "Restricted Repeated Capabilities"="", "Help"="This attribute selects the unit for absolute measurements with a power sensor.\n\nAvailable Repeated Capabilities:\nNone\n\nRemote-control command(s):\nUNIT<1|2>:PMETer:POWer DBM | W", "Flags"={"OPC Wait"=FALSE, "Dont check status"=FALSE, "*WAI"=FALSE}, "Check Status Callback"=""}, {"Level"=3, "Descriptive Name"="PWM Relative Units", "Class Only"=FALSE, "Data Type"=0, "Access"=2, "Identifier"="RSZVL_ATTR_PMET_UNIT_REL", "Range Table"="rszvl_rngPmetUnitRel", "Command"="UNIT:PMET:POW:RAT", "Read Callback"="", "Write Callback"="", "Range Callback"="", "Check Callback"="", "Rngtable Callback"="", "Coerce Callback"="", "User Callback"="", "Supported Models"="", "Instrument Options"="", "Repeated Capabilities"="", "Restricted Repeated Capabilities"="", "Help"="This attribute selects the unit for relative measurements with a power sensor.\n\nAvailable Repeated Capabilities:\nNone\n\nRemote-control command(s):\nUNIT<1|2>:PMETer:POWer:RATio DB | PCT", "Flags"={"OPC Wait"=FALSE, "Dont check status"=FALSE, "*WAI"=FALSE}, "Check Status Callback"=""}, {"Level"=3, "Descriptive Name"="PWM Power Meter State", "Class Only"=FALSE, "Data Type"=3, "Access"=2, "Identifier"="RSZVL_ATTR_PMET_STATE", "Range Table"="", "Command"="SENS:PMET", "Read Callback"="", "Write Callback"="", "Range Callback"="", "Check Callback"="", "Rngtable Callback"="", "Coerce Callback"="", "User
